vi "Pockels Cal-AutoMeasure loop.vi"(6 "Timed out (in)":bool, 7 "Pockels control voltage index":i32, 9 "Abort this objective":refnum<vi>, 10 "Abort":refnum<vi>, 11 "Measured power ind":refnum<vi>) -> (0 "error out":errorcluster, 1 "Abort this objective":bool, 2 "Aborted":bool, 3 "Measured power (mW)":dbl format="%#.4f", 4 "Timed out":bool)   [LabVIEW 2013]
uses:
  <vilib>/DAQmx/read.llb/DAQmx Read (Analog DBL 1Chan 1Samp).vi
  <vilib>/DAQmx/miscellaneous.llb/DAQmx Fill In Error Info.vi
  Globals/gl_Calibration globals.vi
panel:
  in  "Rolling Average window (sec)":i32=10
  in  "Stabilisation time (s)":dbl=2.0 format="%#_13g"
  in  "Maximum timee to wait (s)":dbl=60.0 format="%#_13g"
  out "Weighted COV":dbl format="%#.4f"
  in  "Enable sim":bool
  in  "Sim":dbl(knob) scale=-1.0..1.0
  out "Raw":dbl format="%#.4f"
  out "Mean power (mW)":dbl format="%#.4f"
  out "COV":dbl format="%#.4f"
  in  "Sim force completion":bool
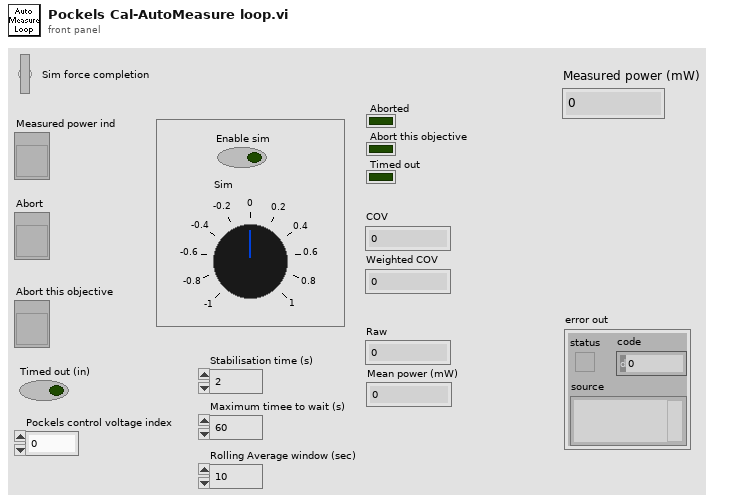
[diagram p1: front panel]
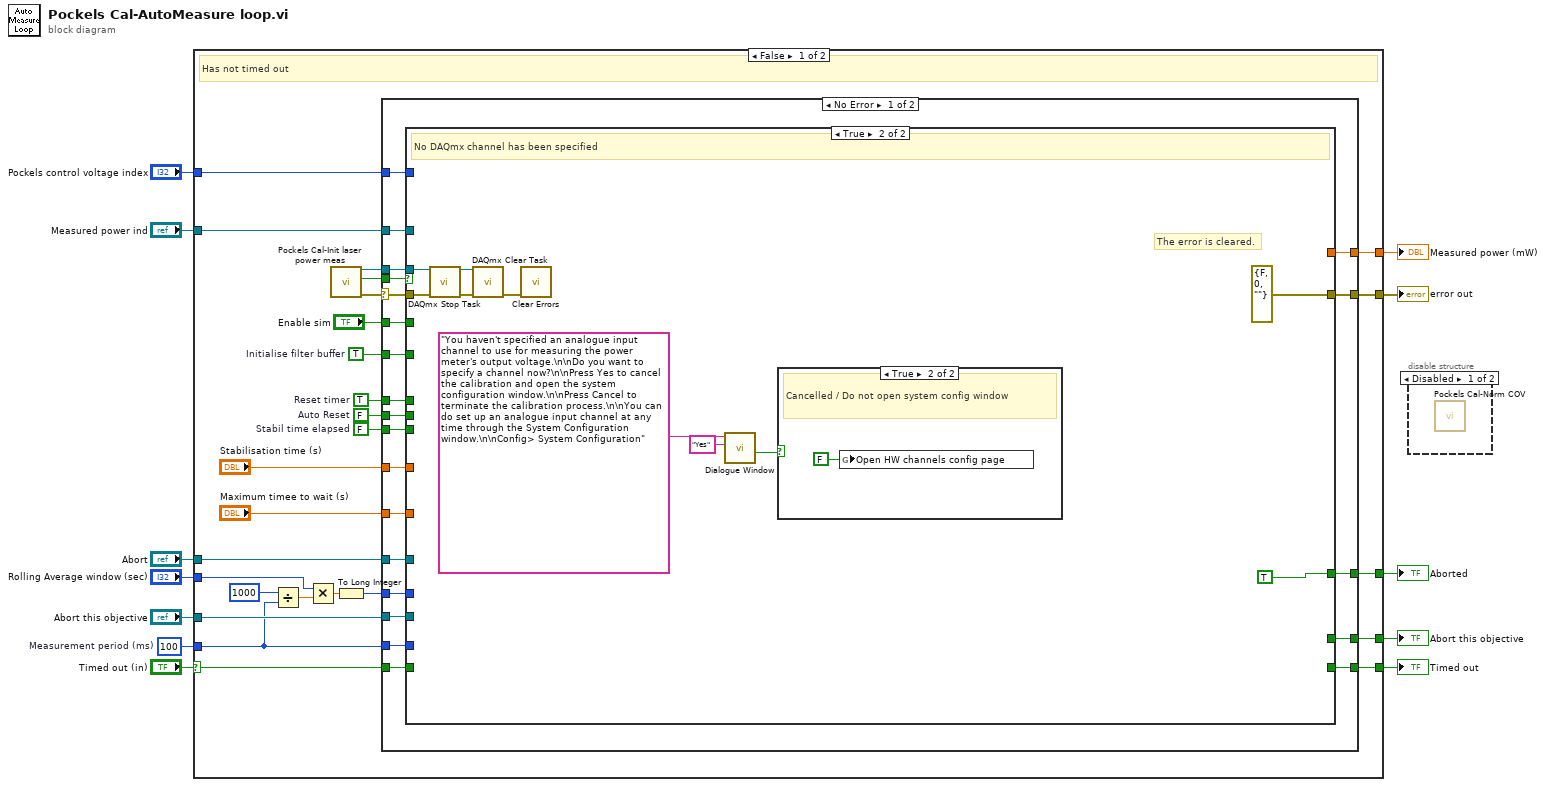
[diagram p0: block diagram]
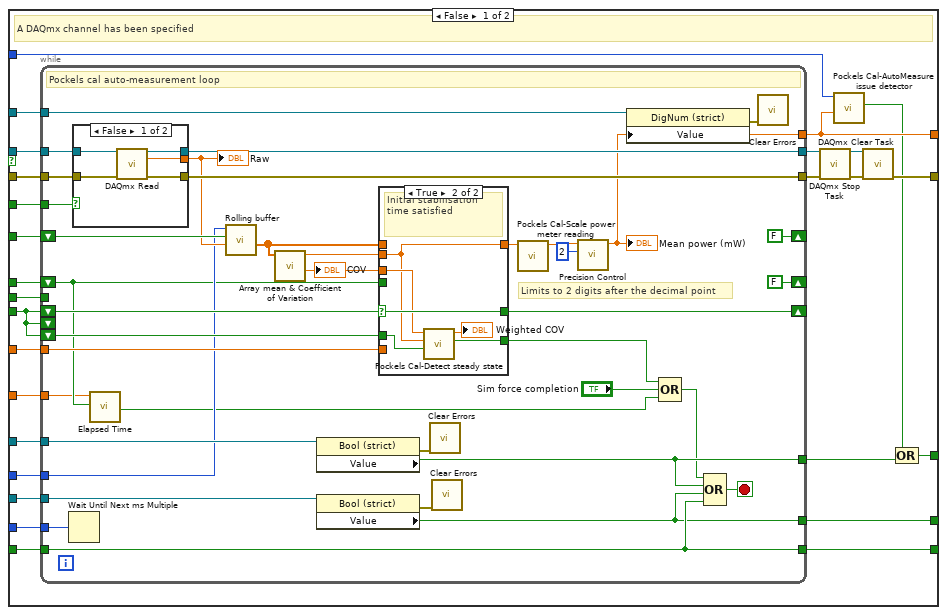
[diagram p3: hidden frame]
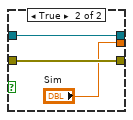
[diagram p4: hidden frame]
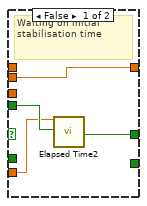
[diagram p5: hidden frame]
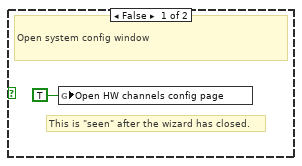
[diagram p6: hidden frame]
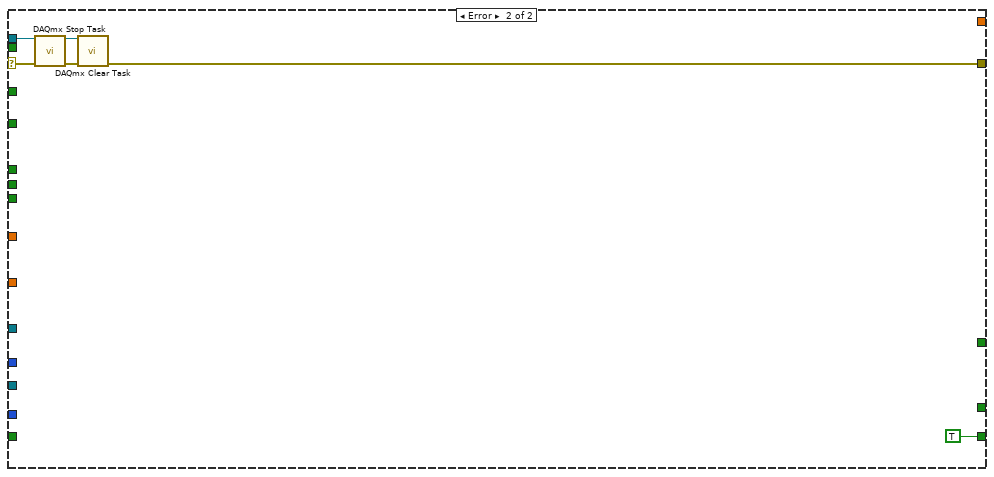
[diagram p7: hidden frame]
diagram:
  w5 = u32 100  # Measurement period (ms)
  n1 = case shown="False" "Timed out (in)" {
    selector: "Timed out (in)" -> [w30 w162]
    tunnel: [w38 _] -> w12
    tunnel: "Abort this objective" -> [w37 _]
    tunnel: "Measured power ind" -> [w36 _]
    tunnel: [w35 _] -> w9
    tunnel: [w34 w162] -> w8
    tunnel: "Abort" -> [w33 _]
    tunnel: [w17 _] -> w3
    tunnel: w5 -> [w24 _]
    tunnel: "Rolling Average window (sec)" -> [w27 _]
    tunnel: [w15 _] -> w2
    tunnel: "Pockels control voltage index" -> [w13 _]
    frame False {
      w18 = TRUE  # Initialise filter buffer
      w21 = FALSE  # Auto Reset
      w22 = FALSE  # Stabil time elapsed
      w23 = TRUE  # Reset timer
      # "Has not timed out"
      n2 = Divide(x=u32 1000, y=w24) -> (x/y=w28:dbl)
      n3 = Multiply(x=w27, y=w28) -> (x*y=w26:dbl)
      n4 = call "Pockels Cal-Init laser power meas.vi"() -> ("error out"=w32:errorcluster, "Auto-cancel"=w16:bool, "Laser power measrement task"=w31:refnum<k21>)  [unwired: 9 in]
      n5 = To Long Integer(number=w26) -> (32bit integer=w25:i32)
      n6 = case shown="No Error" w32 {
        selector: w32 -> [w51 w157]
        tunnel: [w60 _] -> w38
        tunnel: w37 -> [w59 _]
        tunnel: w36 -> [w58 _]
        tunnel: [w57 _] -> w35
        tunnel: w30 -> [w56 _]
        tunnel: [w55 TRUE] -> w34
        tunnel: w33 -> [w54 _]
        tunnel: [w53 _] -> w17
        tunnel: w31 -> [w52 w158]
        tunnel: w24 -> [w50 _]
        tunnel: w25 -> [w49 _]
        tunnel: w23 -> [w48 _]
        tunnel: w22 -> [w45 _]
        tunnel: w21 -> [w47 _]
        tunnel: "Enable sim" -> [w46 _]
        tunnel: "Stabilisation time (s)" -> [w44 _]
        tunnel: w18 -> [w43 _]
        tunnel: w16 -> [w42 _]
        tunnel: [w41 w156] -> w15
        tunnel: "Maximum timee to wait (s)" -> [w40 _]
        tunnel: w13 -> [w39 _]
        frame No Error {
          n7 = case shown="True" w42 {
            tunnel: [w87 _] -> w60
            tunnel: w59 -> [w86 _]
            tunnel: w58 -> [w85 _]
            tunnel: [w63 TRUE ("Value")] -> w57
            tunnel: w56 -> [w84 _]
            tunnel: [w83 _] -> w55
            tunnel: w54 -> [w82 _]
            tunnel: [w65 _] -> w53
            tunnel: w52 -> [w81 w147]
            tunnel: w51 -> [w80 w148]
            tunnel: w50 -> [w79 _]
            tunnel: w49 -> [w78 _]
            tunnel: w48 -> [w77 _]
            tunnel: w47 -> [w76 _]
            tunnel: w46 -> [w75 _]
            tunnel: w45 -> [w74 _]
            tunnel: w44 -> [w73 _]
            tunnel: w43 -> [w72 _]
            tunnel: [w67 errorcluster {"status"=FALSE, "code"=0, "source"=""} ("error out")] -> w41
            tunnel: w40 -> [w66 _]
            tunnel: w39 -> [w64 _]
            frame False {
              # "A DAQmx channel has been specified"
              n8 = while {
                tunnel: w82 -> [w125]
                tunnel: [w121] -> w83
                tunnel: w84 -> [w121]
                tunnel: [w124] -> w62
                tunnel: w85 -> [w122]
                tunnel: w86 -> [w120]
                tunnel: [w119] -> w87
                tunnel: [w88] -> w65
                tunnel: w81 -> [w118]
                tunnel: [w117] -> w68
                tunnel: [w108] -> w69
                tunnel: w80 -> [w116]
                tunnel: w79 -> [w115]
                tunnel: w78 -> [w99]
                shift-right: [FALSE ("Reset timer")] -> _
                shift-left: w77 -> [w92]
                shift-right: [w113] -> _
                shift-left: w74 -> [w112]
                tunnel: w76 -> [_]
                tunnel: w75 -> [w107]
                shift-left: w74 -> [_]
                shift-left: w74 -> [w106]
                tunnel: w73 -> [w103]
                shift-right: [FALSE ("Initialise filter buffer")] -> _
                shift-left: w72 -> [w101]
                tunnel: w66 -> [w91]
                stop <- w123 stop-if-true
                # "Limits to 2 digits after the decimal point"
                # "Pockels cal auto-measurement loop"
                n9 = Wait Until Next ms Multiple(millisecond multiple=w115) -> ()  [unwired: 1 out]
                n10 = case shown="False" w107 {
                  tunnel: w118 -> [w130 w133]
                  tunnel: [w129 w132] -> w117
                  tunnel: w116 -> [w128 w132]
                  tunnel: [w127 "Sim"] -> w100
                  tunnel: [w126 w133] -> w108
                  frame False {
                    n11 = call-poly <vilib>:"DAQmx Read.vi"("task/channels in"=w130, "error in"=w128) -> ("task out"=w126:refnum<k21>, "data"=w127:dbl, "error out"=w129:errorcluster)  [unwired: 11 in]
                  }
                  frame True {
                  }
                }
                "Raw" <- w100
                n12 = call "Elapsed Time"("Time Target (s)"=w91, "Reset"=w92) -> ("Time has Elapsed"=w89:bool)  [unwired: 10 in, 7 out]
                n13 = call "Rolling buffer.vi"("Value in"=w100, "Reset buffer"=w101, "Buffer length (points)"=w99) -> ("Rolling buffer"=w98:dbl[])  [unwired: 8 in]
                n14 = call "Array mean & Coefficient of Variation.vi"("Data"=w98) -> ("Coeffecient of variation"=w96:dbl, "Mean"=w97:dbl)  [unwired: 9 in]
                "COV" <- w96
                n15 = property class="Bool (strict)"(reference=w125) -> (error out=w111:errorcluster, "Value"=w124:bool)  [unwired: 1 in, 1 out]
                n16 = property class="Bool (strict)"(reference=w120) -> (error out=w109:errorcluster, "Value"=w119:bool)  [unwired: 1 in, 1 out]
                n17 = case shown="True" w112 {
                  selector: w112 -> [_ w143]
                  tunnel: [w134 w138] -> w95
                  tunnel: [w136 w143] -> w113
                  tunnel: w92 -> [w137 _]
                  tunnel: w106 -> [_ w142]
                  tunnel: [_ w141] -> w105
                  tunnel: w103 -> [w135 _]
                  tunnel: w98 -> [_ _]
                  tunnel: w96 -> [_ w139]
                  tunnel: w97 -> [w134 w138]
                  frame False {
                    # "Waiting on initial stabilisation time"
                    n18 = call "Elapsed Time2"("Time Target (s)"=w135, "Reset"=w137) -> ("Time has Elapsed"=w136:bool)  [unwired: 10 in, 7 out]
                  }
                  frame True {
                    # "Initial stabilisation time satisfied"
                    n19 = call "Pockels Cal-Detect steady state.vi"("Stabil time elapsed"=w142, "Average V"=w138, "Coeffecient of variation"=w139) -> ("Steady state?"=w141:bool, "Weighted COV"=→"Weighted COV":dbl)  [unwired: 7 in]
                  }
                }
                n20 = call <vilib>:"Clear Errors.vi"("error in (no error)"=w111) -> ()  [unwired: 6 in, 1 out]
                n21 = call <vilib>:"Clear Errors.vi"("error in (no error)"=w109) -> ()  [unwired: 6 in, 1 out]
                n22 = call "Pockels Cal-Scale power meter reading.vi"("Power meter measured voltage (V)"=w95) -> ("Power meter measured power (mW)"=w94:dbl)  [unwired: 10 in]
                n23 = call "Precision Control.vi"("Precision"=u8 2, "Input Value"=w94) -> ("Output Value"=w88:dbl)  [unwired: 8 in, 1 out]
                "Mean power (mW)" <- w88
                n24 = property class="DigNum (strict)"(reference=w122, "Value"=w88) -> (error out=w110:errorcluster)  [unwired: 1 in, 1 out]
                n25 = Compound Arithmetic op=OR(w105, "Sim force completion", w89) -> (w90:bool)
                n26 = Compound Arithmetic op=OR(w90, w124, w119, w121) -> (w123:bool)
                n27 = call <vilib>:"Clear Errors.vi"("error in (no error)"=w110) -> ()  [unwired: 6 in, 1 out]
              }
              n28 = call <vilib>:"DAQmx Stop Task.vi"("task/channels in"=w69, "error in"=w68) -> ("task out"=w71:refnum<k21>, "error out"=w70:errorcluster)  [unwired: 12 in]
              n29 = call "Pockels Cal-AutoMeasure issue detector.vi"("New Value (mW)"=w65, "Pockels control voltage index"=w64) -> ("Aborted by the user on detected issue"=w61:bool)  [unwired: 9 in]
              n30 = call <vilib>:"DAQmx Clear Task.vi"("task in"=w71, "error in"=w70) -> ("error out"=w67:errorcluster)  [unwired: 13 in]
              n31 = Compound Arithmetic op=OR(w61, w62) -> (w63:bool)
            }
            frame True {
              # "The error is cleared."
              # "No DAQmx channel has been specified"
              n32 = call <vilib>:"DAQmx Stop Task.vi"("task/channels in"=w147, "error in"=w148) -> ("task out"=w144:refnum<k21>, "error out"=w149:errorcluster)  [unwired: 12 in]
              n33 = call <vilib>:"DAQmx Clear Task.vi"("task in"=w144, "error in"=w149) -> ("error out"=w145:errorcluster)  [unwired: 13 in]
              n34 = call <vilib>:"Clear Errors.vi"("error in (no error)"=w145) -> ()  [unwired: 6 in, 1 out]
              n35 = call "Dialogue Window.vi"("Caption-Right button (OK)"="Yes", "Message string"="You haven't specified an analogue input channel to use for measuring the power meter's output voltage.\n\nDo you want to specify a channel now?\n\nPress Yes to cancel the calibration and open the system configuration window.\n\nPress Cancel to terminate the calibration process.\n\nYou can do set up an analogue input channel at any time through the System Configuration window.\n\nConfig> System Configuration") -> ("Cancelled (Left button pressed)"=w150:bool)  [unwired: 7 in, 2 out]
              n36 = case shown="True" w150 {
                frame False {
                  # "This is \"seen\" after the wizard has closed."
                  # "Open system config window"
                  n37 = global write "gl_Calibration globals.vi" "Open HW channels config page"(TRUE ("Open HW channels config page")) -> ()
                }
                frame True {
                  # "Cancelled / Do not open system config window"
                  n38 = global write "gl_Calibration globals.vi" "Open HW channels config page"(FALSE ("Open HW channels config page")) -> ()
                }
              }
            }
          }
        }
        frame Error {
          n39 = call <vilib>:"DAQmx Stop Task.vi"("task/channels in"=w158, "error in"=w157) -> ("task out"=w160:refnum<k21>, "error out"=w159:errorcluster)  [unwired: 12 in]
          n40 = call <vilib>:"DAQmx Clear Task.vi"("task in"=w160, "error in"=w159) -> ("error out"=w156:errorcluster)  [unwired: 13 in]
        }
      }
    }
    frame True {
      # "Timed out"
    }
  }
  "Abort this objective" <- w12
  "Measured power (mW)" <- w3
  "Aborted" <- w9
  "Timed out" <- w8
  "error out" <- w2
  n41 = disable-structure shown="Disabled" {
    frame Disabled {
      n42 = call "Pockels Cal-Norm COV.vi"() -> ()  [unwired: 11 in, 1 out]
    }
    frame Enabled {
    }
  }
